vi "RSZVB Get Reference Frequency.vi"(8 "error in (no error)":errorcluster {"code" format="%.0x"}, 11 "VISA session":refnum<visa-resource-name>) -> (0 "error out":errorcluster {"code" format="%.0x"}, 2 "Reference Frequency":dbl format="%^.3e", 3 "dup VISA session":refnum<visa-resource-name>)   [LabVIEW 2011]
doc: "This VI queries the frequency of the external reference oscillator.\n\nNote(s):\n\n(1) The frequency must be 10 MHz.\n\nRemote-control command(s):\n[SENSe<Ch>:]ROSCillator:EXTernal:FREQuency?"
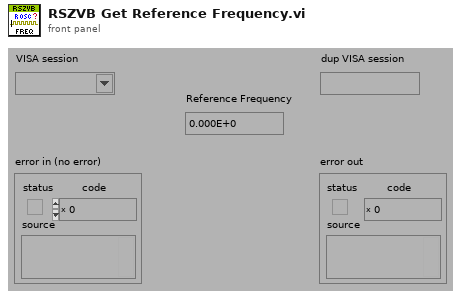
[diagram p1: front panel]
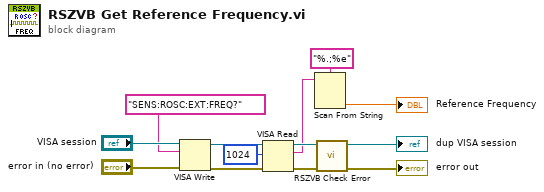
[diagram p0: block diagram]
diagram:
  n1 = VISA Write(VISA resource name="VISA session", write buffer="SENS:ROSC:EXT:FREQ?", error in (no error)="error in (no error)") -> (VISA resource name out=w9:refnum<visa-resource-name>, error out=w10:errorcluster)  [unwired: 1 out]
  n2 = VISA Read(VISA resource name=w9, byte count=u32 1024 ("byte count (0)"), error in (no error)=w10) -> (VISA resource name out=w13:refnum<visa-resource-name>, read buffer=w1:string, error out=w12:errorcluster)  [unwired: 1 out]
  n3 = Scan From String(format string="%.;%e", input string=w1) -> (output 1=→"Reference Frequency":dbl)  [unwired: 3 in, 3 out]
  n4 = call "RSZVB Check Error.vi"("error in (no error)"=w12, "VISA session"=w13) -> ("error out"=→"error out":errorcluster, "dup VISA session"=→"dup VISA session":refnum<visa-resource-name>)  [unwired: 8 in]
